vi "File is not executable--error.vi"() -> (0 "error out":errorcluster)   [LabVIEW 2025]
doc: "Indicates that the specified file exists but does not have extension \"EXE\"."
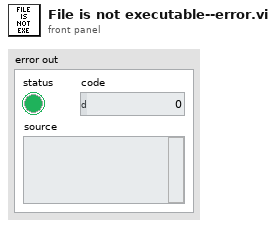
[diagram p1: front panel]
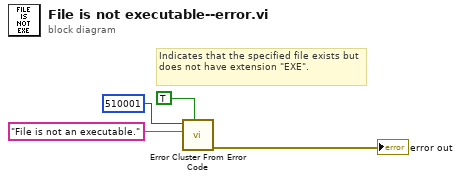
[diagram p0: block diagram]
diagram:
  # "Indicates that the specified file exists but does not have extension \"EXE\"."
  n1 = call <vilib>:"Error Cluster From Error Code.vi"("show call chain? (False)"=TRUE, "error message (\"\")"="File is not an executable." ("error message (\"\")"), "error code (0)"=510001) -> ("error out"=→"error out":errorcluster)  [unwired: 6 in]
